vi "Data DVR to Signal DVR.vi"(8 "error in (no error)":errorcluster, 11 "TreeNode Signal Data":refnum<data-value>) -> (0 "error out":errorcluster, 2 "Signal DVR out":refnum<data-value>, 3 "TreeNode Signal Data Out":refnum<data-value>)   [LabVIEW 2012, in "MDSplus.lvlib" / "Signal.lvclass"]
doc: "Convert Data DVR retrieved from TreeNode Get Data to a Signal DVR to be used by the Signal.lvclass VI's\n\nMB"
uses:
  <vilib>/MDSplus/Classes/Data_Class/Compound_Class/Signal_Class/Signal.lvclass
  <vilib>/MDSplus/Classes/Data_Class/Data.lvclass
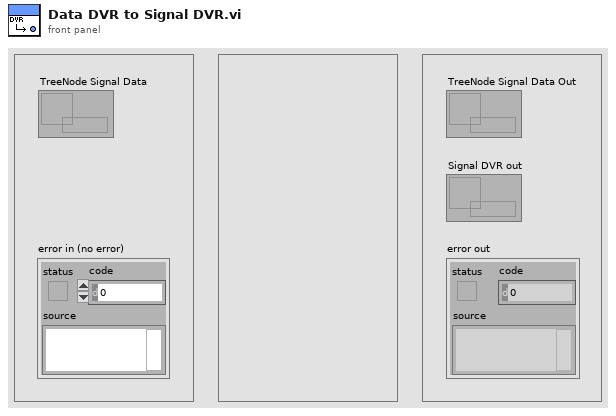
[diagram p1: front panel]
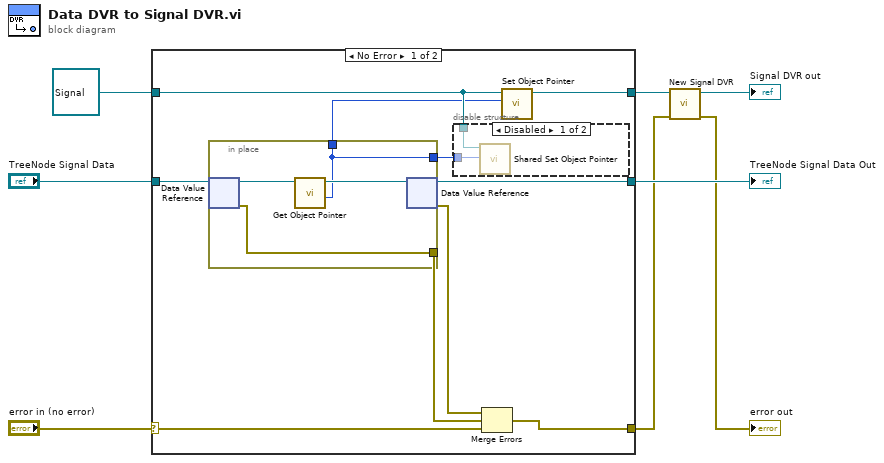
[diagram p0: block diagram]
diagram:
  n1 = case shown="No Error" "error in (no error)" {
    selector: "error in (no error)" -> [w15 w26]
    tunnel: [w10 w27] -> w4
    tunnel: refnum<class "Signal.lvclass"> refnum ("Range in") -> [w11 w27]
    tunnel: [w14 w26] -> w2
    tunnel: "TreeNode Signal Data" -> [w18 w25]
    tunnel: [w13 w25] -> w5
    frame No Error {
      n2 = in-place {
        in-place-border: [w21] -> w12
        in-place-border: [w24] -> w17
        in-place-border: [w21] -> w9
        n3 = in-place-dvr #1(w18) -> (w23:refnum<class "Data.lvclass">, w24:errorcluster)
        n4 = call-dynamic "Get Object Pointer.vi"("Data in"=w23) -> ("Object Pointer"=w21:i64, "Data out"=w22:refnum<class "Data.lvclass">)  [unwired: 8 in, 1 out]
        n5 = in-place-dvr #1(w22) -> (w13:refnum<data-value>, w16:errorcluster)
      }
      n6 = disable-structure shown="Disabled" {
        disable-tunnel: w12 -> [w20 _]
        disable-tunnel: w11 -> [w19 _]
        frame Disabled {
          n7 = call <vilib>:"Shared Set Object Pointer.vi"("Object Pointer"=w20, "Data in"=w19) -> ()  [unwired: 9 in, 1 out]
        }
        frame Enabled {
        }
      }
      n8 = Merge Errors(w16, w17, w15) -> (w14:errorcluster)
      n9 = call-dynamic "Set Object Pointer.vi"("Object Pointer"=w9, "Data in"=w11) -> ("Data out"=w10:refnum<class "Signal.lvclass">)  [unwired: 9 in]
    }
    frame Error {
    }
  }
  "TreeNode Signal Data Out" <- w5
  n10 = call <vilib>:"New Signal DVR.vi"("error in (no error)"=w2, "Signal in"=w4) -> ("error out"=→"error out":errorcluster, "Signal DVR out"=→"Signal DVR out":refnum<data-value>)  [unwired: 8 in]
